vi "While Loop Skip Count.vi"() -> ()   [LabVIEW 2019]
panel:
  out "Result":dbl
  in  "Count by:":dbl
  # "Challenge:\nSkip Count. Count to 100 by twos, threes--whatever number you wish. The program takes an input number and counts by multiples of that number, starting at zero. When the sequence passes 100, the count stops."
  # "Try it: Enter a number in the \"Count by\" box and hit Run."
  # "You will probably need:\nWhile loops, controls and indicators, wait for ms,, comparisons"
  # "Open the block diagram to see a possible solution."
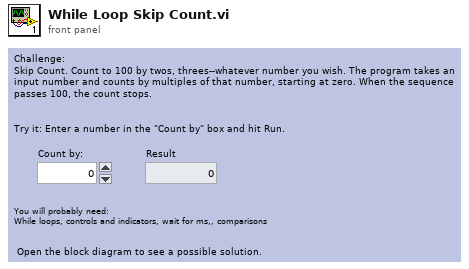
[diagram p1: front panel]
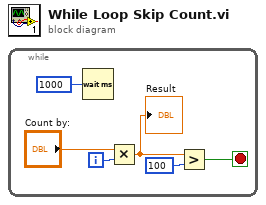
[diagram p0: block diagram]
diagram:
  n1 = while {
    i -> [w5]
    stop <- w1 stop-if-true
    n2 = Wait (ms)(milliseconds to wait=1000) -> ()  [unwired: 1 out]
    n3 = Multiply(x="Count by:", y=w5) -> (x*y=w3:dbl)
    "Result" <- w3
    n4 = Greater?(x=w3, y=100) -> (0:w1:bool)
  }
